vi "deco_ee_568.vi"(4 "data IN":string) -> (0 "TITULOS DIG 9-16":T1, 1 "TITULOS DIG 1-8":T1, 2 "Eeprom":T2 {"Analogicas 32"."?" items=["1", "2", "4", "8", "16", "32", "64", "128", "256"]; "Analogicas 32"."?" items=["Lineal"=15, "Cuadrática"=14]; "Analogicas 32"."unsigned byte array[0]" items=["10000", "1000", "100", "10", "8000", "800", "80", "8", "4000", "400", "40", "4", "2000", "200", "20", "2"]; "Analogicas 16"."?" items=["1", "2", "4", "8", "16", "32", "64", "128", "256"]; "Analogicas 16"."?" items=["Lineal"=15, "Cuadrática"=14]; "Analogicas 16"."unsigned byte array[0]" items=["10000", "1000", "100", "10", "8000", "800", "80", "8", "4000", "400", "40", "4", "2000", "200", "20", "2"]})   [LabVIEW 2010]
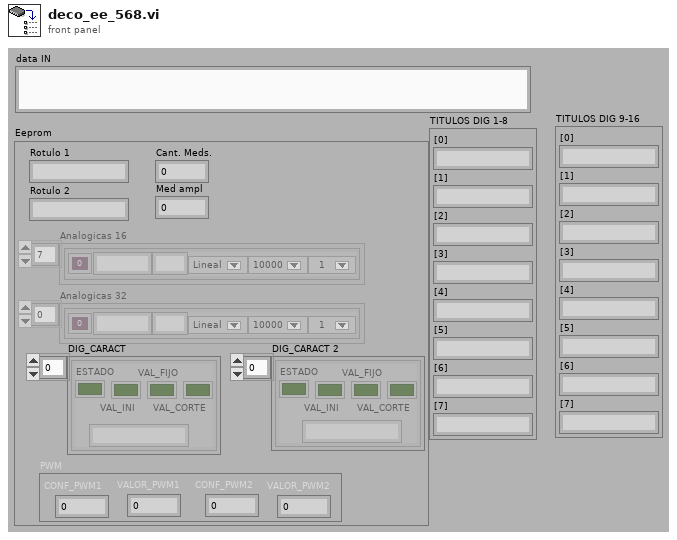
[diagram p1: front panel]
types:
  T1 = cluster{"[0]":string, "[1]":string, "[2]":string, "[3]":string, "[4]":string, "[5]":string, "[6]":string, "[7]":string}
  T2 = cluster{"Rotulo 1":string, "Rotulo 2":string, "Cant. Meds.":u8, "Med ampl":u8, "Analogicas 16":cluster{i32, "mapaeeprom":string, "mapaeeprom":string, u8, "unsigned byte array[0]":u8, u8}[], "Analogicas 32":cluster{i32, "mapaeeprom":string, "mapaeeprom":string, u8, "unsigned byte array[0]":u8, u8}[], "DIG_CARACT":cluster{"ESTADO":bool, "VAL_INI":bool, "VAL_FIJO":bool, "VAL_CORTE":bool, "CARACT LOG 9-16":string}[], "DIG_CARACT 2":cluster{"ESTADO":bool, "VAL_INI":bool, "VAL_FIJO":bool, "VAL_CORTE":bool, "CARACT LOG 9-16":string}[], "PWM":cluster{"CONF_PWM1":u8, "VALOR_PWM1":u8, "CONF_PWM2":u8, "VALOR_PWM2":u8}}
  T3 = cluster{"unsigned byte array[0]":u8, "unsigned byte array[1]":u8, "unsigned byte array[2]":u8, "unsigned byte array[3]":u8}
  T4 = cluster{bool, bool, bool, bool, "data IN":string}
  T5 = cluster{i32, "data IN":string, "data IN":string, u8, u8, "unsigned byte array[0]":u8}
  T6 = cluster{i32, "data IN":string, "data IN":string, u8, u8, "unsigned byte array[0]":u8}[]
  T7 = cluster{"data IN":string, "data IN":string, u8, u8, cluster{i32, "data IN":string, "data IN":string, u8, u8, "unsigned byte array[0]":u8}[], cluster{i32, "data IN":string, "data IN":string, u8, u8, "unsigned byte array[0]":u8}[], cluster{bool, bool, bool, bool, "data IN":string}[], cluster{bool, bool, bool, bool, "data IN":string}[], "unsigned byte array":cluster{"unsigned byte array[0]":u8, "unsigned byte array[1]":u8, "unsigned byte array[2]":u8, "unsigned byte array[3]":u8}}
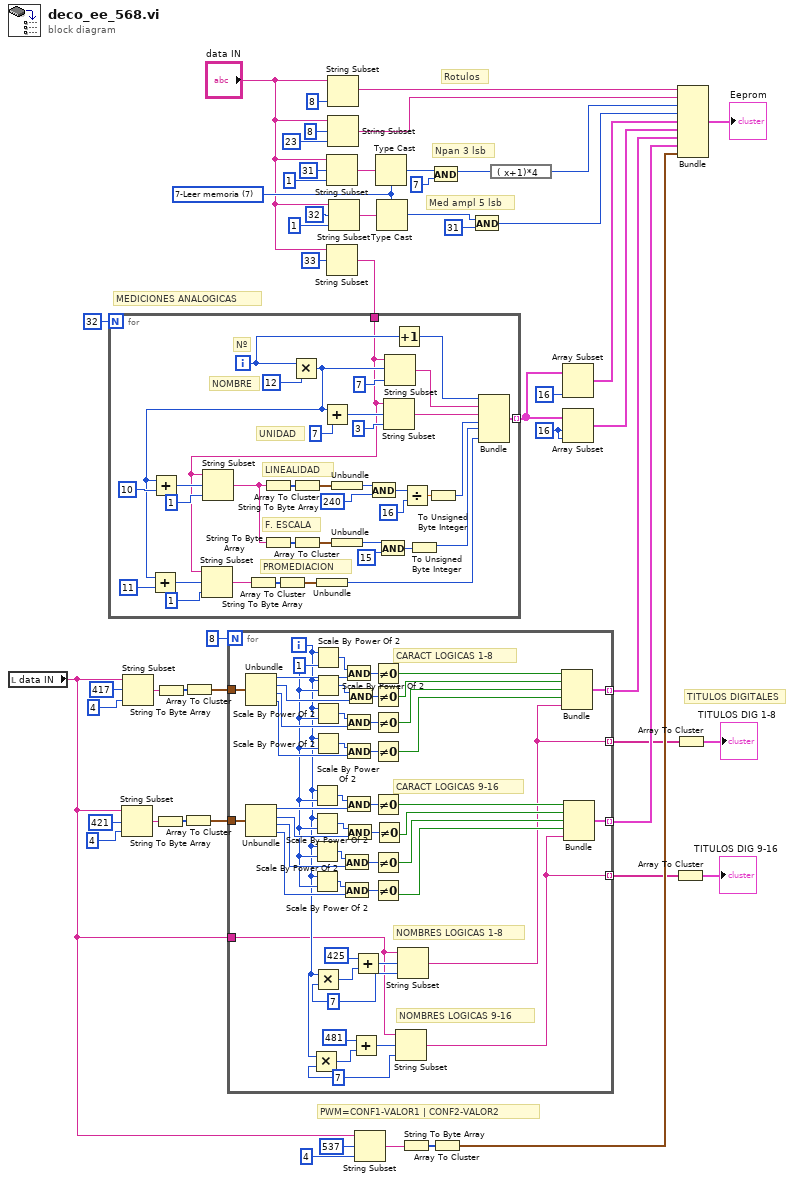
[diagram p0: block diagram]
diagram:
  w7 = 16 ("index")
  w52 = u8 7 items=["1-Leer Página"=1, "2-Subir página"=2, "3-Bajar Página"=3, "4-Leer Datos "=4, "5-Digital Write"=5, "6-Digital Write c/mascara"=6, "7-Leer memoria"=7, "8-Escribe memoria"=8, "9-Leer PWM1/2"=16, "10-Escribir PWM1/2"=17] ("Comando: 2")
  # "TITULOS DIGITALES"
  # "PWM=CONF1-VALOR1 | CONF2-VALOR2"
  # "MEDICIONES ANALOGICAS"
  # "Med ampl 5 lsb"
  # "Npan 3 lsb"
  # "Rotulos"
  n1 = local read "data IN"() -> (w14:string)
  n2 = String Subset(string=w14, offset (0)=421, length (rest)=4 ("length (rest)")) -> (substring=w17:string)
  n3 = String Subset(string=w14, offset (0)=417, length (rest)=4 ("length (rest)")) -> (substring=w23:string)
  n4 = String To Byte Array(string=w17) -> (unsigned byte array=w18:u8[])
  n5 = String To Byte Array(string=w23) -> (unsigned byte array=w22:u8[])
  n6 = Array To Cluster(array=w18) -> (cluster=w15:T3)
  n7 = Array To Cluster(array=w22) -> (cluster=w20:T3)
  n8 = for {
    N: 8 -> [_]
    tunnel: [w101] -> w6 mode=indexing
    tunnel: [w68] -> w5 mode=indexing
    tunnel: w20 -> [w67]
    tunnel: w15 -> [w66]
    tunnel: w14 -> [w55]
    tunnel: [w54] -> w2 mode=indexing
    tunnel: [w53] -> w1 mode=indexing
    i -> [w56]
    w60 = 7 ("length (rest)")
    w61 = 7 ("length (rest)")
    w65 = u8 1 ("x")
    # "NOMBRES LOGICAS 9-16"
    # "NOMBRES LOGICAS 1-8"
    # "CARACT LOGICAS 1-8"
    # "CARACT LOGICAS 9-16"
    n9 = Unbundle(w67) -> ("unsigned byte array[0]"=w88:u8, "unsigned byte array[1]"=w87:u8, "unsigned byte array[2]"=w86:u8, "unsigned byte array[3]"=w85:u8)
    n10 = Unbundle(w66) -> ("unsigned byte array[0]"=w81:u8, "unsigned byte array[1]"=w82:u8, "unsigned byte array[2]"=w83:u8, "unsigned byte array[3]"=w84:u8)
    n11 = Multiply(x=w56, y=w60) -> (x*y=w57:i32)
    n12 = Scale By Power Of 2(n=w56, x=w65) -> (x*2^n=w70:u8)
    n13 = Scale By Power Of 2(n=w56, x=w65) -> (x*2^n=w71:u8)
    n14 = Scale By Power Of 2(n=w56, x=w65) -> (x*2^n=w74:u8)
    n15 = Scale By Power Of 2(n=w56, x=w65) -> (x*2^n=w75:u8)
    n16 = Scale By Power Of 2(n=w56, x=w65) -> (x*2^n=w99:u8)
    n17 = Scale By Power Of 2(n=w56, x=w65) -> (x*2^n=w98:u8)
    n18 = Scale By Power Of 2(n=w56, x=w65) -> (x*2^n=w95:u8)
    n19 = Scale By Power Of 2(n=w56, x=w65) -> (x*2^n=w94:u8)
    n20 = Multiply(x=w56, y=w61) -> (x*y=w64:i32)
    n21 = And(x=w74, y=w83) -> (x .and. y?=w73:u8)
    n22 = And(x=w75, y=w84) -> (x .and. y?=w76:u8)
    n23 = And(x=w99, y=w88) -> (x .and. y?=w100:u8)
    n24 = And(x=w95, y=w86) -> (x .and. y?=w96:u8)
    n25 = And(x=w94, y=w85) -> (x .and. y?=w93:u8)
    n26 = And(x=w70, y=w81) -> (x .and. y?=w69:u8)
    n27 = And(x=w71, y=w82) -> (x .and. y?=w72:u8)
    n28 = And(x=w98, y=w87) -> (x .and. y?=w97:u8)
    n29 = Add(x=481 ("offset (0)"), y=w57) -> (x+y=w59:i32)
    n30 = Add(x=425 ("offset (0)"), y=w64) -> (x+y=w62:i32)
    n31 = Not Equal To 0?(x=w100) -> (x != 0?=w92:bool)
    n32 = Not Equal To 0?(x=w97) -> (x != 0?=w91:bool)
    n33 = Not Equal To 0?(x=w96) -> (x != 0?=w90:bool)
    n34 = Not Equal To 0?(x=w93) -> (x != 0?=w89:bool)
    n35 = Not Equal To 0?(x=w69) -> (x != 0?=w77:bool)
    n36 = Not Equal To 0?(x=w73) -> (x != 0?=w79:bool)
    n37 = Not Equal To 0?(x=w76) -> (x != 0?=w80:bool)
    n38 = Not Equal To 0?(x=w72) -> (x != 0?=w78:bool)
    n39 = String Subset(string=w55, offset (0)=w59, length (rest)=w60) -> (substring=w53:string)
    n40 = String Subset(string=w55, offset (0)=w62, length (rest)=w61) -> (substring=w54:string)
    n41 = Bundle(w92, w91, w90, w89, "data IN"=w54) -> (w101:T4)  [unwired: 1 in]
    n42 = Bundle(w77, w78, w79, w80, "data IN"=w53) -> (w68:T4)  [unwired: 1 in]
  }
  n43 = String Subset(string="data IN", offset (0)=31, length (rest)=1 ("length (rest)")) -> (substring=w47:string)
  n44 = String Subset(string="data IN", offset (0)=33) -> (substring=w51:string)  [unwired: 1 in]
  n45 = for {
    N: 32 -> [_]
    tunnel: w51 -> [w106]
    tunnel: [w104] -> w30 mode=indexing
    i -> [w133]
    # "PROMEDIACION"
    # "F. ESCALA"
    # "LINEALIDAD"
    # "NOMBRE"
    # "UNIDAD"
    # "Nº"
    n46 = Multiply(x=w133, y=12 ("offset (0)")) -> (x*y=w107:i32)
    n47 = Add(x=w107, y=11) -> (x+y=w114:i32)
    n48 = Add(x=w107, y=10) -> (x+y=w129:i32)
    n49 = String Subset(string=w106, offset (0)=w114, length (rest)=1 ("length (rest)")) -> (substring=w110:string)
    n50 = String Subset(string=w106, offset (0)=w129, length (rest)=1 ("length (rest)")) -> (substring=w122:string)
    n51 = String To Byte Array(string=w110) -> (unsigned byte array=w112:u8[])
    n52 = String To Byte Array(string=w122) -> (unsigned byte array=w127:u8[])
    n53 = String To Byte Array(string=w122) -> (unsigned byte array=w124:u8[])
    n54 = Array To Cluster(array=w112) -> (cluster=w111:cluster{"unsigned byte array[0]":u8})
    n55 = Array To Cluster(array=w127) -> (cluster=w126:cluster{"unsigned byte array[0]":u8})
    n56 = Array To Cluster(array=w124) -> (cluster=w125:cluster{"unsigned byte array[0]":u8})
    n57 = Unbundle(w111) -> ("unsigned byte array[0]"=w109:u8)
    n58 = Add(x=w107, y=7) -> (x+y=w135:i32)
    n59 = Unbundle(w126) -> ("unsigned byte array[0]"=w119:u8)
    n60 = Unbundle(w125) -> ("unsigned byte array[0]"=w121:u8)
    n61 = And(x=w119, y=u8 240 ("value")) -> (x .and. y?=w117:u8)
    n62 = And(x=w121, y=u8 15 ("value")) -> (x .and. y?=w116:u8)
    n63 = String Subset(string=w106, offset (0)=w135, length (rest)=3 ("length (rest)")) -> (substring=w131:string)
    n64 = String Subset(string=w106, offset (0)=w107, length (rest)=7 ("length (rest)")) -> (substring=w132:string)
    n65 = Increment(x=w133) -> (x+1=w105:i32)
    n66 = Divide(x=w117, y=i8 16) -> (x/y=w102:dbl)
    n67 = To Unsigned Byte Integer(number=w116) -> (unsigned 8bit integer=w108:u8)
    n68 = To Unsigned Byte Integer(number=w102) -> (unsigned 8bit integer=w103:u8)
    n69 = Bundle(w105, "data IN"=w132, "data IN"=w131, w103, w108, "unsigned byte array[0]"=w109) -> (w104:T5)  [unwired: 1 in]
  }
  n70 = String Subset(string="data IN", length (rest)=8 ("length (rest)")) -> (substring=w45:string)  [unwired: 1 in]
  n71 = String Subset(string="data IN", offset (0)=8, length (rest)=23 ("length (rest)")) -> (substring=w46:string)
  n72 = String Subset(string="data IN", offset (0)=32, length (rest)=1 ("length (rest)")) -> (substring=w48:string)
  n73 = String Subset(string=w14, offset (0)=537, length (rest)=4 ("length (rest)")) -> (substring=w12:string)
  n74 = Type Cast(type=w52, x=w47) -> (*(type *) &x=w37:u8)
  n75 = Type Cast(type=w52, x=w48) -> (*(type *) &x=w33:u8)
  n76 = String To Byte Array(string=w12) -> (unsigned byte array=w13:u8[])
  n77 = And(x=w37, y=u8 7) -> (x .and. y?=w10:u8)
  n78 = Array To Cluster(array=w13) -> (cluster=w11:T3)
  n79 = And(x=w33, y=u8 31) -> (x .and. y?=w34:u8)
  n80 = expression code="( x+1)*4"(w10) -> (w9:u8)
  n81 = Array Subset(array=w30, length=16) -> (w29:T6)  [unwired: 1 in]
  n82 = Array Subset(array=w30, index=w7, length=w7) -> (w31:T6)
  n83 = Array To Cluster(array=w1) -> (cluster=→"TITULOS DIG 9-16":T1)
  n84 = Array To Cluster(array=w2) -> (cluster=→"TITULOS DIG 1-8":T1)
  n85 = Bundle("data IN"=w45, "data IN"=w46, w9, w34, w29, w31, w6, w5, "unsigned byte array"=w11) -> (→"Eeprom":T7)  [unwired: 1 in]
